vi "Create SSL BIO from Socket Object.vi"(8 "error in (no error)":errorcluster, 10 "TCP Object":u64, 11 "SSL-Context in":refnum<class "SSL Context.lvclass">) -> (0 "error out":errorcluster, 3 "BIO out":refnum<class "BIO.lvclass">)   [LabVIEW 2013, in "OpenSSL Socket.lvlib" / "SSL Socket.lvclass"]
doc: "Binds a TCP socket descriptor to an SSL BIO object."
uses:
  SSL Socket.lvclass
  SSL Context/SSL Context.lvclass
  SSL_Lib/BIO/BIO.lvclass
  SSL_Lib/SSL/SSL_Mode.ctl
  SSL Context/SSL Context.lvclass/SSL Context.ctl
  SSL Context/Read SSL Context.vi
  SSL_Lib/SSL-Context/SSL-Context.lvclass
  SSL_Lib/SSL/SSL.lvclass
  SSL_Lib/SSL-Lib/SSL-Lib.lvclass
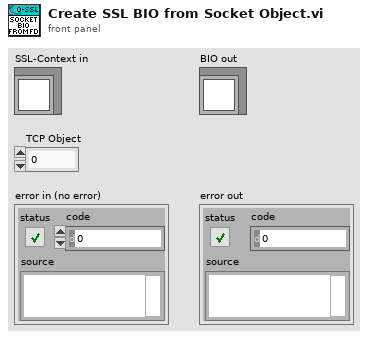
[diagram p1: front panel]
types:
  T1 = typedef "OpenSSL Socket.lvlib/SSL.lvclass/SSL_Mode.ctl" = i32
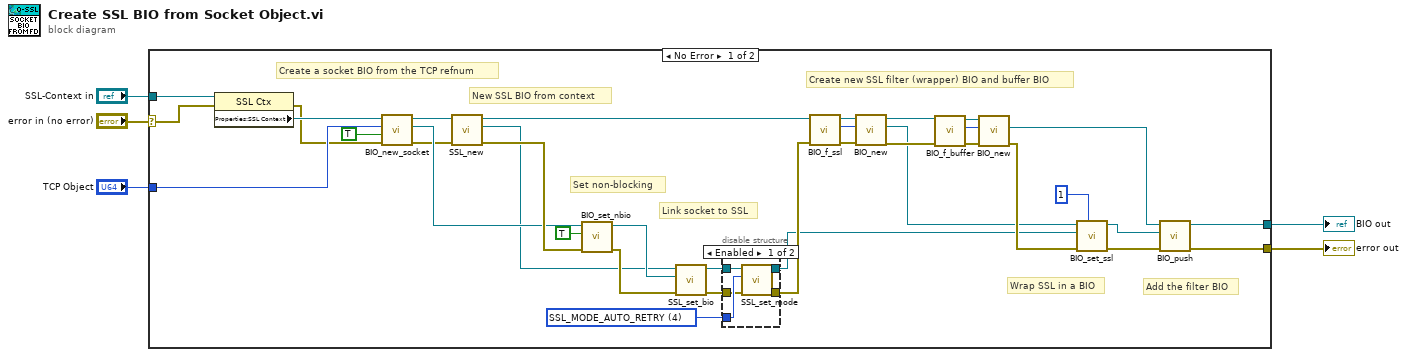
[diagram p0: block diagram]
diagram:
  n1 = case shown="No Error" "error in (no error)" {
    selector: "error in (no error)" -> [w6 w49]
    tunnel: "TCP Object" -> [w33 _]
    tunnel: [w32 _] -> w4
    tunnel: [w31 w49] -> w3
    tunnel: "SSL-Context in" -> [w9 _]
    frame No Error {
      w10 = T1 4 items=["None"=0, "SSL_MODE_ENABLE_PARTIAL_WRITE"=1, "SSL_MODE_ACCEPT_MOVING_WRITE_BUFFER"=2, "SSL_MODE_AUTO_RETRY"=4, "SSL_MODE_RELEASE_BUFFERS"=16, "SSL_MODE_SEND_FALLBACK_SCSV"=128] ("Mode")
      # "Add the filter BIO"
      # "Wrap SSL in a BIO"
      # "Create new SSL filter (wrapper) BIO and buffer BIO"
      # "Link socket to SSL"
      # "Set non-blocking"
      # "New SSL BIO from context"
      # "Create a socket BIO from the TCP refnum"
      n2 = property class="SSL Ctx"(reference=w9, error in=w6) -> (error out=w7:errorcluster, "Properties:SSL Context"=w8:refnum<class "SSL-Context.lvclass">)  [unwired: 1 out]
      n3 = call "BIO_new_socket.vi"("error in (no error)"=w7, "Close on free? (T)"=TRUE, "fd"=w33, "SSL-Context in"=w8) -> ("error out"=w13:errorcluster, "Socket BIO out"=w16:refnum<class "BIO.lvclass">, "SSL-Context out"=w14:refnum<class "SSL-Context.lvclass">)  [unwired: 5 in]
      n4 = call "SSL_new.vi"("error in (no error)"=w13, "SSL-Context in"=w14) -> ("error out"=w19:errorcluster, "SSL out"=w15:refnum<class "SSL.lvclass">, "SSL-Context out"=w36:refnum<class "SSL-Context.lvclass">)  [unwired: 7 in]
      n5 = call "BIO_set_nbio.vi"("error in (no error)"=w19, "Non-Blocking?"=TRUE, "BIO in"=w16) -> ("error out"=w41:errorcluster, "BIO out"=w18:refnum<class "BIO.lvclass">)  [unwired: 7 in]
      n6 = call "SSL_set_bio.vi"("error in (no error)"=w41, "BIO"=w18, "SSL in"=w15) -> ("error out"=w20:errorcluster, "SSL out"=w17:refnum<class "SSL.lvclass">)  [unwired: 7 in]
      n7 = disable-structure shown="Enabled" {
        disable-tunnel: w10 -> [w46 _]
        disable-tunnel: w17 -> [w45 w48]
        disable-tunnel: w20 -> [w44 w47]
        disable-tunnel: [w43 w48] -> w37
        disable-tunnel: [w42 w47] -> w38
        frame Enabled {
          n8 = call "SSL_set_mode.vi"("error in (no error)"=w44, "Mode"=w46, "SSL in"=w45) -> ("error out"=w42:errorcluster, "SSL out"=w43:refnum<class "SSL.lvclass">)  [unwired: 7 in]
        }
        frame Disabled {
        }
      }
      n9 = call "BIO_f_ssl.vi"("error in (no error)"=w38, "SSL-Lib in"=w36) -> ("error out"=w24:errorcluster, "*BIO_Method"=w26:u64, "SSL-Lib out"=w25:refnum<class "SSL-Context.lvclass">)  [unwired: 7 in]
      n10 = call "BIO_new.vi"("error in (no error)"=w24, "*BIO_method"=w26, "SSL-Lib in"=w25) -> ("error out"=w35:errorcluster, "BIO out"=w27:refnum<class "BIO.lvclass">, "SSL-Lib out"=w39:refnum<class "SSL-Context.lvclass">)  [unwired: 6 in]
      n11 = call "BIO_f_buffer.vi"("error in (no error)"=w35, "SSL-Lib in"=w39) -> ("error out"=w21:errorcluster, "*BIO_Method"=w23:u64, "SSL-Lib out"=w22:refnum<class "SSL-Context.lvclass">)  [unwired: 7 in]
      n12 = call "BIO_new.vi"("error in (no error)"=w21, "*BIO_method"=w23, "SSL-Lib in"=w22) -> ("error out"=w40:errorcluster, "BIO out"=w29:refnum<class "BIO.lvclass">)  [unwired: 6 in, 1 out]
      n13 = call "BIO_set_ssl.vi"("close flag"=1, "error in (no error)"=w40, "SSL in"=w37, "BIO in"=w27) -> ("error out"=w34:errorcluster, "BIO out"=w30:refnum<class "BIO.lvclass">)  [unwired: 6 in]
      n14 = call "BIO_push.vi"("error in (no error)"=w34, "New BIO"=w30, "BIO in"=w29) -> ("error out"=w31:errorcluster, "BIO out"=w32:refnum<class "BIO.lvclass">)  [unwired: 7 in]
    }
    frame Error {
    }
  }
  "BIO out" <- w4
  "error out" <- w3
